vi "Sine_Formula.vi"() -> ()   [LabVIEW 2024]
panel:
  in  "input variable":dbl
  out "output variable":dbl
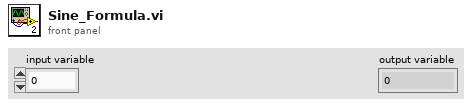
[diagram p1: front panel]
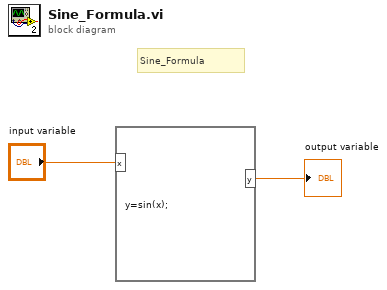
[diagram p0: block diagram]
diagram:
  # "Sine_Formula"
  n1 = formula code="y=sin(x);"("x"="input variable") -> ("y"=→"output variable":dbl)
